vi "Set Up Objects.vi"(8 "error in (no error)":errorcluster, 10 "len":dbl, 11 "Height Map":dbl[][](array[numeric])) -> (0 "error out":errorcluster, 3 "Main Scene Object Ref (out)":refnum<vi>)   [LabVIEW 2023]
doc: "Creates the root scene object."
uses:
  <vilib>/picture/picture.llb/imagedata.ctl
  <vilib>/picture/3D Picture Control/Object/Create Object (drawable).vi
  <vilib>/picture/3D Picture Control/Helpers/Apply Texture (no reference).vi
  <vilib>/picture/3D Picture Control/Object/Create Object (name).vi
  <vilib>/picture/3D Picture Control/Object/Add Object (no reference).vi
  <vilib>/picture/3D Picture Control/NI_3D Picture Control.lvlib
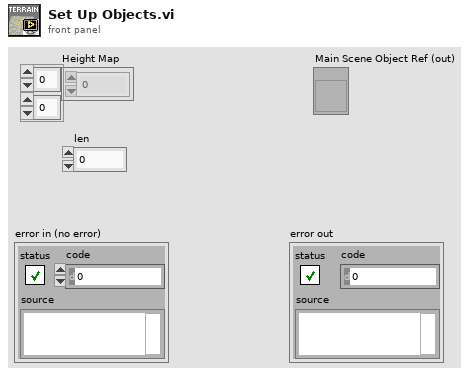
[diagram p1: front panel]
types:
  T1 = typedef "imagedata.ctl" = cluster{"image type":i32, "image depth":i32, "image":u8[], "mask":u8[], "colors":u32[], "Rectangle":cluster{"left":i16, "top":i16, "right":i16, "bottom":i16}}
  T2 = enum16{"As a Decal", "With Modulation", "With Blending", "As a replacement"}
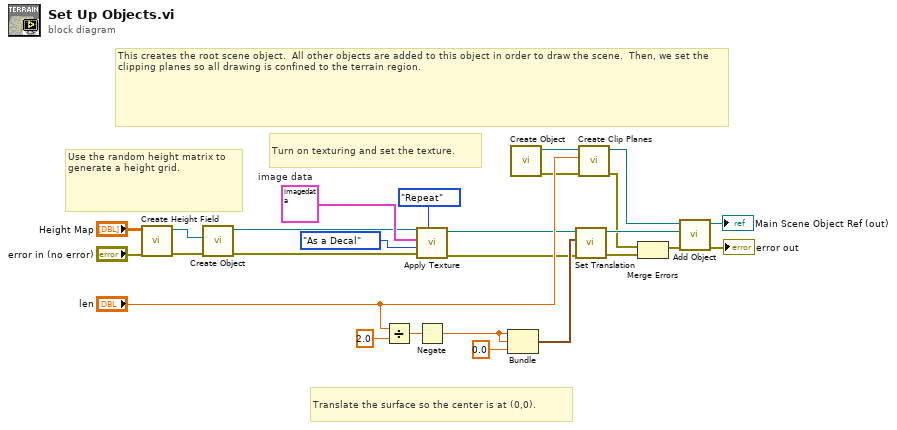
[diagram p0: block diagram]
diagram:
  w16 = T1 {"image type"=0, "image depth"=24, "image"=array[1500000 elements], "mask"=[], "colors"=[], "Rectangle"={"left"=0, "top"=0, "right"=1000, "bottom"=500}}  # image data
  # "This creates the root scene object.  All other objects are added to this object in order to draw the scene.  Then, we set the clipping planes so all drawing is confined to the terrain region."
  # "Translate the surface so the center is at (0,0)."
  # "Turn on texturing and set the texture."
  # "Use the random height matrix to generate a height grid."
  n1 = call <vilib>:"Create Height Field.vi"("error in (no error)"="error in (no error)", "Data"="Height Map") -> ("error out"=w17:errorcluster, "New Height Field Refnum"=w18:refnum<vi>)  [unwired: 2 in, 6 out]
  n2 = call-poly <vilib>:"Create Object.vi"("error in (no error)"=w17, "Geometry"=w18) -> ("error out"=w8:errorcluster, "Scene:New Object"=w13:refnum<vi>)  [unwired: 8 in]
  n3 = Divide(x="len", y=2.0 ("x")) -> (x/y=w23:dbl)
  n4 = call-poly <vilib>:"Apply Texture.vi"("Horizontal Wrap Mode"=enum16{"Clamp", "Repeat"}."Repeat", "error in (no error)"=w8, "Apply Mode"=T2."As a Decal", "Image Data"=w16, "Scene Object In"=w13) -> ("error out"=w3:errorcluster, "Scene Object Out"=w12:refnum<vi>)  [unwired: 5 in]
  n5 = Negate(x=w23) -> (-x=w20:dbl)
  n6 = Bundle(w20, w20, "-x"=0.0) -> (w22:cluster{dbl, dbl, "-x":dbl})  [unwired: 1 out]
  n7 = call-poly <vilib>:"Create Object.vi"() -> ("error out"=w4:errorcluster, "Scene:New Object"=w25:refnum<vi>)  [unwired: 10 in]
  n8 = call <vilib>:"Set Translation.vi"("error in (no error)"=w3, "Translation"=w22, "Scene Object"=w12) -> ("error out"=w7:errorcluster, "Translated Object"=w10:refnum<vi>)  [unwired: 7 out]
  n9 = call "Create Clip Planes.vi"("error in (no error)"=w4, "Terrain Size"="len", "Main Scene Object Ref"=w25) -> ("error out"=w5:errorcluster, "Main Scene Object Ref (out)"=w11:refnum<vi>)  [unwired: 7 out]
  n10 = Merge Errors(w5, w7) -> (w6:errorcluster)
  n11 = call-poly <vilib>:"Add Object.vi"("error in (no error)"=w6, "New Object In"=w10, "Scene Object In"=w11) -> ("error out"=→"error out":errorcluster, "Scene Object Out"=→"Main Scene Object Ref (out)":refnum<vi>)  [unwired: 7 in]
